vi "Delay progress bar.vi"(8 "error in (no error)":errorcluster, 10 "Title Message":string="Waiting countdown bar", 11 "delay time mecs":u32) -> (0 "error out":errorcluster)   [LabVIEW 2024]
panel:
  out "Numeric 2":sgl format="%.2f"
  out "Numeric":sgl format="%.2f"
  out "?":i32(slide) max=10000 scale=0.0..20000.0
  # "seconds left to wait"
  # "OF"
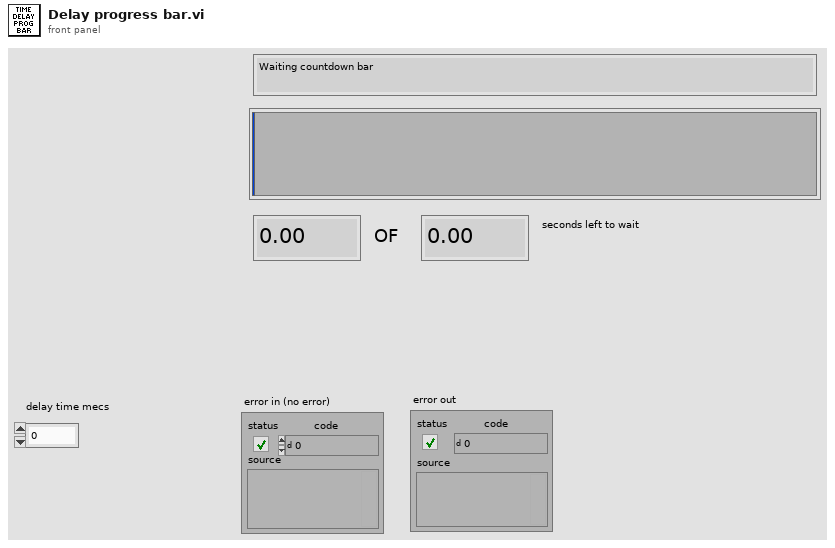
[diagram p1: front panel]
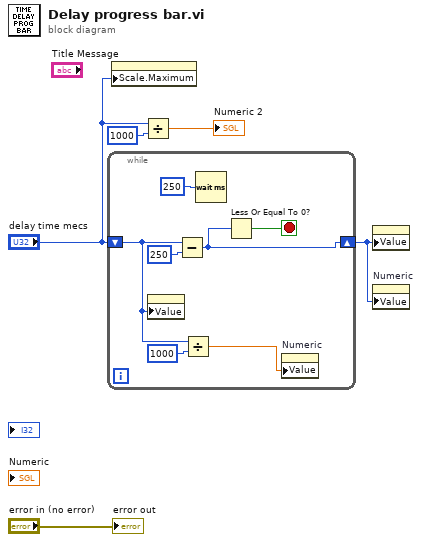
[diagram p0: block diagram]
diagram:
  n1 = while {
    shift-right: [w9] -> w4
    shift-left: "delay time mecs" -> [w8]
    stop <- w10 stop-if-true
    n2 = property class="Slide (strict)"("Value"=w8) -> ()  [unwired: 2 in, 2 out]
    n3 = Subtract(x=w8, y=u32 250) -> (x-y=w9:u32)
    n4 = Divide(x=w8, y=u32 1000) -> (x/y=w6:dbl)
    n5 = Wait (ms)(milliseconds to wait=u32 250) -> ()  [unwired: 1 out]
    n6 = Less Or Equal To 0?(x=w9) -> (x <= 0?=w10:bool)
    n7 = property on="Numeric" class="DigNum (strict)"("Value"=w6) -> ()  [unwired: 2 in, 2 out]
  }
  n8 = property class="Slide (strict)"("Scale.Maximum"="delay time mecs") -> ()  [unwired: 2 in, 2 out]
  n9 = Divide(x="delay time mecs", y=u32 1000) -> (x/y=→"Numeric 2":dbl)
  n10 = property class="Slide (strict)"("Value"=w4) -> ()  [unwired: 2 in, 2 out]
  n11 = property on="Numeric" class="DigNum (strict)"("Value"=w4) -> ()  [unwired: 2 in, 2 out]
  "error out" <- "error in (no error)"
